vi "Extract TTL Indices.vi"(3 "Analog TTL":dbl[](array[numeric])) -> (0 "Falling Transition Indices":u32[](array[numeric]), 1 "Rising Transition Indices":u32[](array[numeric]))   [LabVIEW 2009]
uses:
  <vilib>/Waveform/DTblOps.llb/DTbl Analog to Digital.vi
panel:
  out "subarray":u32[](array[numeric])
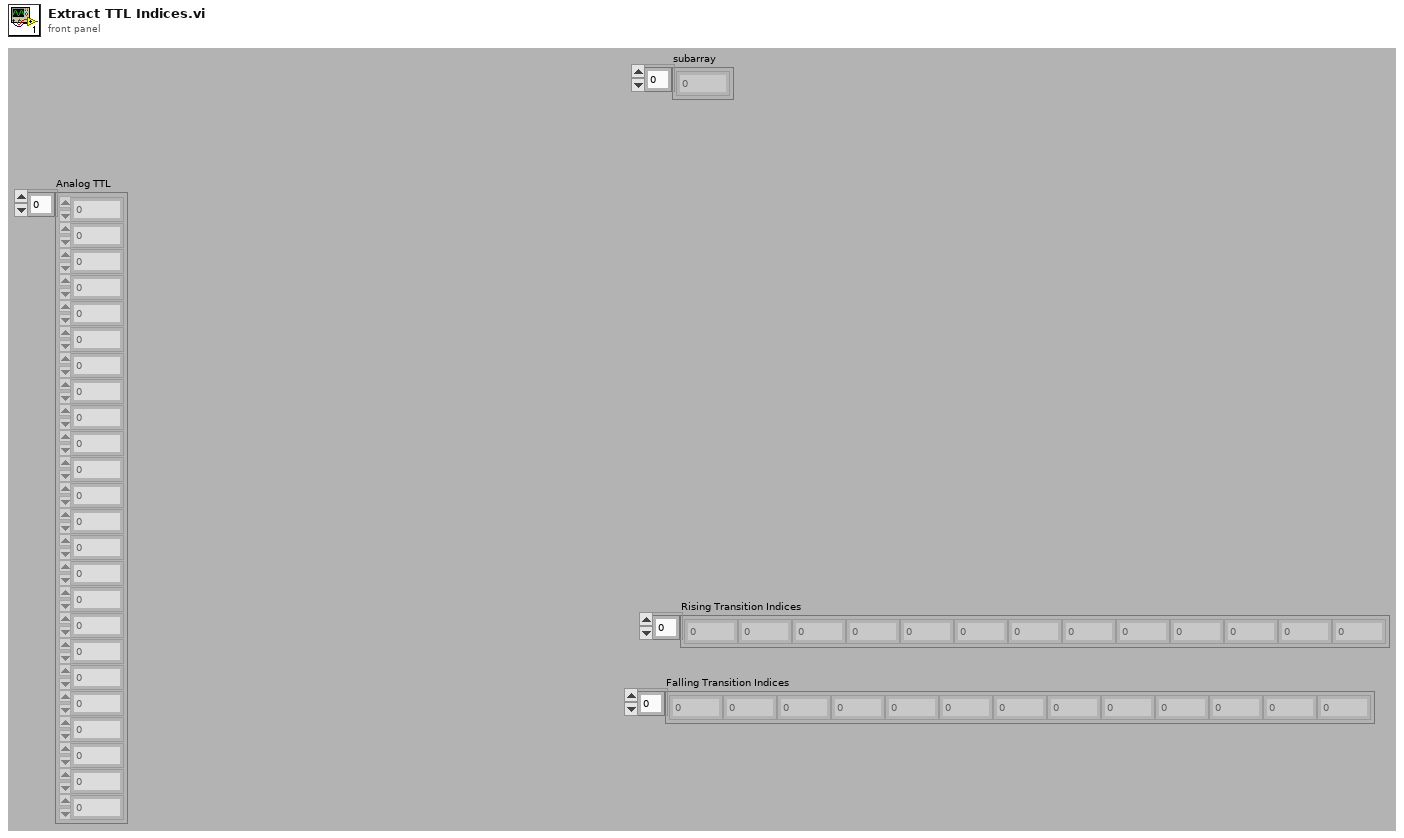
[diagram p1: front panel]
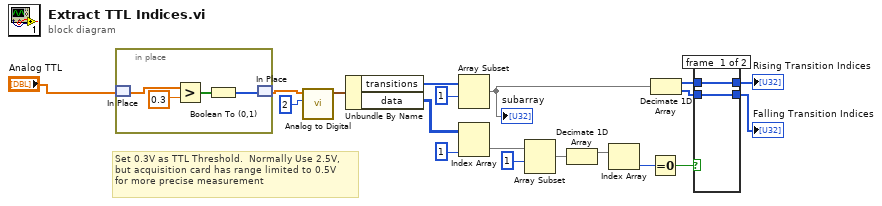
[diagram p0: block diagram]
diagram:
  # "Set 0.3V as TTL Threshold.  Normally Use 2.5V,\nbut acquisition card has range limited to 0.5V \nfor more precise measurement"
  n1 = in-place {
    n2 = in-place-match #1("Analog TTL") -> (w21:dbl[])
    n3 = Greater?(x=w21, y=0.3) -> (0:w23:bool[])
    n4 = Boolean To (0,1)(Boolean=w23) -> (0, 1=w20:i16[])
    n5 = in-place-match #1(w20) -> (w1:dbl[])
  }
  n6 = call-poly <vilib>:"Analog to Digital.vi"("resolution (16 bit)"=2, "analog waveform"=w1) -> ("digital data"=w18:digitaldata)  [unwired: 6 in, 3 out]
  n7 = Unbundle By Name(w18) -> ("transitions"=w8:u32[], "data"=w17:u8[][])
  n8 = Array Subset(array=w8, index=1) -> (w6:u32[])  [unwired: 1 in]
  "subarray" <- w6
  n9 = Index Array(array=w17, index (col)=1 ("disabled index (col)")) -> (element=w5:u8[])  [unwired: 1 in]
  n10 = Array Subset(array=w5, index=1) -> (w4:u8[])  [unwired: 1 in]
  n11 = Decimate 1D Array(w4) -> (w15:u8[])  [unwired: 1 out]
  n12 = Index Array(array=w15) -> (element=w14:u8)  [unwired: 1 in]
  n13 = Equal To 0?(x=w14) -> (x = 0?=w13:bool)
  n14 = Decimate 1D Array(w6) -> (w12:u32[], w9:u32[])
  n15 = case shown="True" w13 {
    tunnel: w12 -> [w25 w27]
    tunnel: w9 -> [w24 w26]
    tunnel: [w24 w27] -> w10
    tunnel: [w25 w26] -> w11
    frame #0 {
    }
    frame #1 {
    }
  }
  "Rising Transition Indices" <- w11
  "Falling Transition Indices" <- w10
